vi "Generate Change Page Event.vi"(8 "error in (no error)":errorcluster, 9 "Target Page":T1=enum."Input Info", 11 "Source Page":T1=enum."Input Info") -> (0 "error out":errorcluster)   [LabVIEW 2020, in "WebServiceImporter.lvlib" / "Main Panel.lvlib" / "Events.lvlib"]
uses:
  <vilib>/Platform/WebService/Main Panel/Events/Events.lvlib
  <vilib>/Platform/WebService/Main Panel/Events/Data Type/Page.ctl
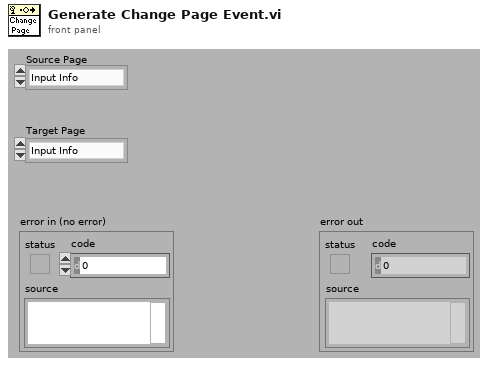
[diagram p1: front panel]
types:
  T1 = typedef "WebServiceImporter.lvlib/Main Panel.lvlib/Events.lvlib/Page.ctl" = enum16{"Input WSDL", "Input Authentication", "Input Info", "Select Methods", "Preview", "Progress", "Finish"}
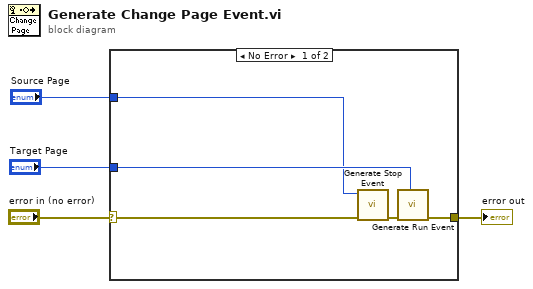
[diagram p0: block diagram]
diagram:
  n1 = case shown="No Error" "error in (no error)" {
    selector: "error in (no error)" -> [w9 w10]
    tunnel: [w6 w10] -> w3
    tunnel: "Source Page" -> [w5 _]
    tunnel: "Target Page" -> [w7 _]
    frame No Error {
      n2 = call <vilib>:"Generate Stop Event.vi"("error in (no error)"=w9, "Page"=w5) -> ("error out"=w8:errorcluster)  [unwired: 9 in]
      n3 = call <vilib>:"Generate Run Event.vi"("error in (no error)"=w8, "Page"=w7) -> ("error out"=w6:errorcluster)  [unwired: 9 in]
    }
    frame Error {
    }
  }
  "error out" <- w3
